vi "FPGA Globals.vi"() -> ()   [LabVIEW 2017]
panel:
  out "Tach Event2?":bool
  out "Tach Event1?":bool
  out "Tach Event0?":bool
  in  "OversampleClk Ticks":u32
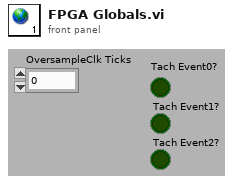
[diagram p1: front panel]
diagram:
